vi "SCP Upload File.vi"(8 "Error In":errorcluster, 9 "Target Directory":string="/home/debian/", 10 "Local File":path, 11 "SCP Session":refnum<k24>) -> (0 "Error Out":errorcluster, 3 "SCP Session":refnum<k24>)   [LabVIEW 2024, in "LMH-LINX.lvlib"]
uses:
  <vilib>/MakerHub/LINX/LMH-LINX.lvlib
  <vilib>/net/SFTP/NI_SFTP.lvlib
  <vilib>/net/SFTP/API/Upload File.vi
  <vilib>/MakerHub/LINX/Private/Utilties/SSH/SSH OpenSSH Session Op.ctl
  <vilib>/MakerHub/LINX/Resources/Renci.SshNet.dll
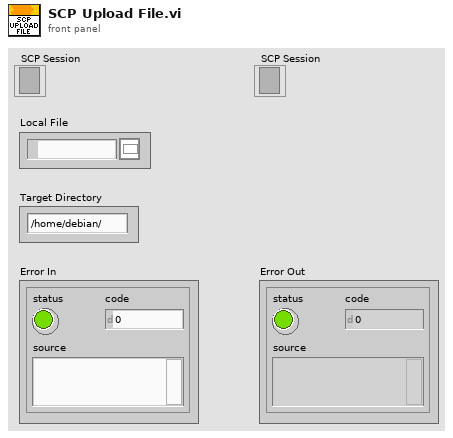
[diagram p1: front panel]
types:
  T1 = typedef "LMH-LINX.lvlib/SSH OpenSSH Session Op.ctl" = enum16{"Get", "Set"}
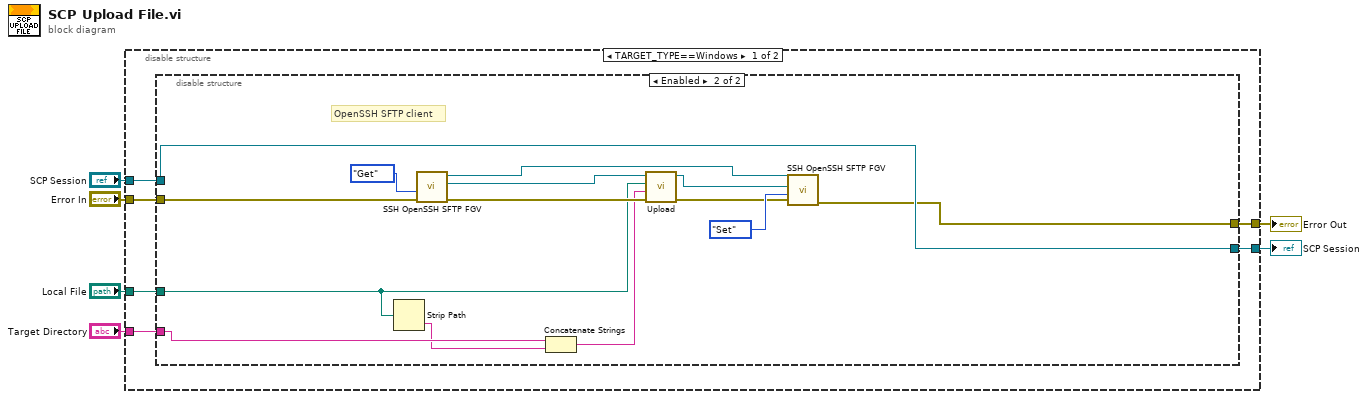
[diagram p0: block diagram]
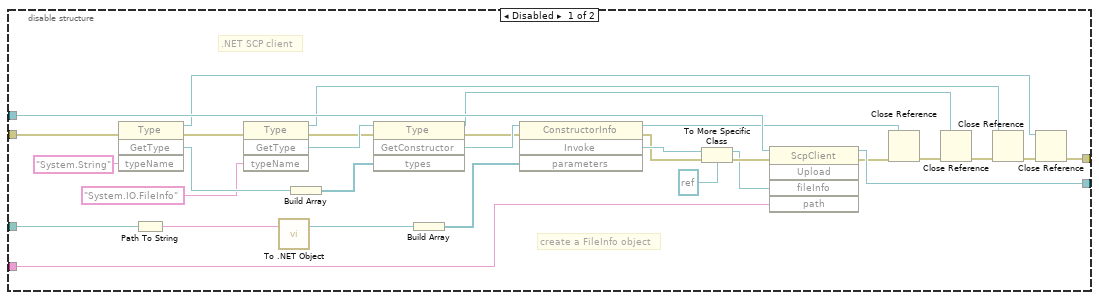
[diagram p2: hidden frame]
diagram:
  n1 = disable-structure shown="TARGET_TYPE==Windows" {
    disable-tunnel: "Local File" -> [w12 _]
    disable-tunnel: "Target Directory" -> [w11 _]
    disable-tunnel: "Error In" -> [w10 _]
    disable-tunnel: [w9 _] -> w3
    disable-tunnel: "SCP Session" -> [w8 _]
    disable-tunnel: [w7 _] -> w1
    frame condition #0 (active) {
      n2 = disable-structure shown="Enabled" {
        disable-tunnel: w12 -> [w42 w52]
        disable-tunnel: w11 -> [w41 w51]
        disable-tunnel: w10 -> [w39 w57]
        disable-tunnel: [w27 w53] -> w9
        disable-tunnel: w8 -> [w26 w53]
        disable-tunnel: [w13 w44] -> w7
        frame Disabled {
          # ".NET SCP client"
          # "create a FileInfo object"
          n3 = invoke class="Type" method="GetType"(error in=w39, "typeName"="System.String") -> (reference out=w14:refnum<k24>, error out=w25:errorcluster, "GetType"=w31:refnum<k24>)  [unwired: 2 in, 1 out]
          n4 = Path To String(path=w42) -> (string=w43:string)
          n5 = invoke class="Type" method="GetType"(error in=w25, "typeName"="System.IO.FileInfo") -> (reference out=w16:refnum<k24>, error out=w24:errorcluster, "GetType"=w29:refnum<k24>)  [unwired: 2 in, 1 out]
          n6 = call <vilib>:"To .NET Object.vi"("anything"=w43) -> (".NET object"=w34:refnum<k24>)  [unwired: 1 in, 1 out]
          n7 = Build Array(w31) -> (w33:refnum<k24>[])
          n8 = invoke class="Type" method="GetConstructor"(reference=w29, error in=w24, "types"=w33) -> (reference out=w17:refnum<k24>, error out=w23:errorcluster, "GetConstructor"=w32:refnum<k24>)  [unwired: 1 in, 1 out]
          n9 = Build Array(w34) -> (w35:refnum<k24>[])
          n10 = invoke class="ConstructorInfo" method="Invoke"(reference=w32, error in=w23, "parameters"=w35) -> (reference out=w20:refnum<k24>, error out=w22:errorcluster, "Invoke"=w37:refnum<k24>)  [unwired: 1 in, 1 out]
          n11 = To More Specific Class(target class=refnum<k24> refnum ("fileInfo"), reference=w37, error in=w22) -> (specific class reference=w38:refnum<k24>, error out=w40:errorcluster)
          n12 = invoke class="ScpClient" method="Upload"(reference=w26, error in=w40, "fileInfo"=w38, "path"=w41) -> (reference out=w27:refnum<k24>, error out=w21:errorcluster)  [unwired: 1 in, 3 out]
          n13 = Close Reference(reference=w20, error in (no error)=w21) -> (error out=w19:errorcluster)
          n14 = Close Reference(reference=w17, error in (no error)=w19) -> (error out=w18:errorcluster)
          n15 = Close Reference(reference=w16, error in (no error)=w18) -> (error out=w15:errorcluster)
          n16 = Close Reference(reference=w14, error in (no error)=w15) -> (error out=w13:errorcluster)
        }
        frame Enabled {
          # "OpenSSH SFTP client"
          n17 = Strip Path(path=w52) -> (name=w50:string)  [unwired: 1 out]
          n18 = call <vilib>:"SSH OpenSSH SFTP FGV.vi"("error in (no error)"=w57, "OpenSSH Session Op"=SSH_OpenSSH_Session_Op."Get") -> ("error out"=w56:errorcluster, "OpenSSH Session out"=w54:refnum<class "Session.lvclass">, "OpenSSH SFTP out"=w46:refnum<class "OpenSSH Client.lvclass">)  [unwired: 7 in]
          n19 = Concatenate Strings(w51, w50) -> (w49:string)
          n20 = call-poly <vilib>:"Upload.vi"("error in"=w56, "remote path"=w49, "local path"=w52, "session in"=w54) -> ("error out"=w47:errorcluster, "session out"=w45:refnum<class "Session.lvclass">)  [unwired: 6 in]
          n21 = call <vilib>:"SSH OpenSSH SFTP FGV.vi"("error in (no error)"=w47, "OpenSSH Session Op"=SSH_OpenSSH_Session_Op."Set", "OpenSSH Session in"=w45, "OpenSSH SFTP in"=w46) -> ("error out"=w44:errorcluster)  [unwired: 5 in, 2 out]
        }
      }
    }
    frame condition #1 {
    }
  }
  "Error Out" <- w1
  "SCP Session" <- w3
